vi "Close.vi"(8 "error in (no error)":errorcluster, 11 "PSP-405 resource in":refnum<visa-resource-name>) -> (0 "error out":errorcluster)   [LabVIEW 2017, in "GW Instek PSP-405.lvlib"]
doc: "Terminates the software connection to the instrument."
uses:
  GW Instek PSP-405.lvlib
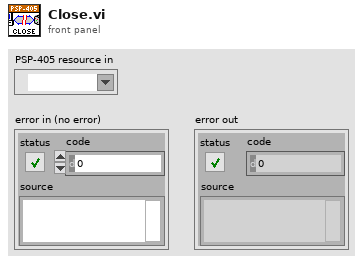
[diagram p1: front panel]
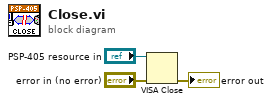
[diagram p0: block diagram]
diagram:
  n1 = VISA Close(VISA resource name="PSP-405 resource in", error in (no error)="error in (no error)") -> (error out=→"error out":errorcluster)
